vi "环境动力接口交互.vi"   [LabVIEW 2016]
uses:
  PLC/PLC.lvlib
types:
  T1 = cluster{"R0":i16, "R1":i16, "R2":i16, "R3":i16, "R4":i16, "R5":i16, "R6":i16, "R7":i16, "R8":i16, "R9":i16, "R10":i16, "R11":i16, "R12":i16, "R13":i16, "R14":i16, "R15":i16, "R16":i16, "R17":i16, "R18":i16, "R19":i16, "R20":i16, "R21":i16, "R22":i16, "R23":i16, "R24":i16, "R25":i16, "R26":i16, "R27":i16, "R28":i16, "R29":i16, "R30":i16, "R31":i16, "R32":i16, "R33":i16, "R34":i16, "R35":i16, "R36":i16, "R37":i16, "R38":i16, "R39":i16}
  T2 = cluster{"R100":i16, "R101":i16, "R102":i16, "R103":i16, "R104":i16, "R105":i16, "R106":i16, "R107":i16, "R108":i16, "R109":i16, "R110":i16, "R111":i16, "R112":i16, "R113":i16, "R114":i16, "R115":i16, "R116":i16, "R117":i16, "R118":i16, "R119":i16, "R120":i16, "R121":i16, "R122":i16, "R123":i16}
  T3 = cluster{"AD0":sgl, "AD1":sgl, "AD2":sgl, "AD3":sgl, "AD4":sgl, "AD5":sgl}
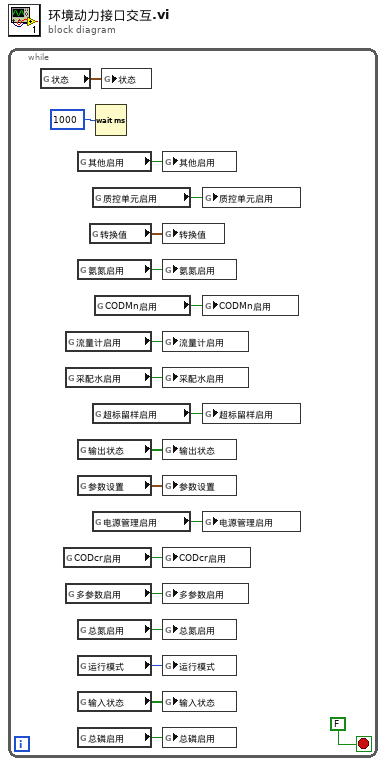
[diagram p0: block diagram]
diagram:
  n1 = while {
    stop <- FALSE stop-if-true
    n2 = global read "采配水全局变量.vi" "状态"() -> (w8:T1)
    n3 = global read "系统设置全局变量.vi" "CODcr启用"() -> (w17:bool)
    n4 = global read "系统设置全局变量.vi" "流量计启用"() -> (w5:bool)
    n5 = global read "系统设置全局变量.vi" "采配水启用"() -> (w15:bool)
    n6 = global read "系统设置全局变量.vi" "多参数启用"() -> (w3:bool)
    n7 = global read "系统设置全局变量.vi" "其他启用"() -> (w4:bool)
    n8 = global read "系统设置全局变量.vi" "氨氮启用"() -> (w16:bool)
    n9 = global read "采配水全局变量.vi" "输出状态"() -> (w20:bool[])
    n10 = global read "采配水全局变量.vi" "参数设置"() -> (w13:T2)
    n11 = global read "系统设置全局变量.vi" "总氮启用"() -> (w11:bool)
    n12 = global read "系统设置全局变量.vi" "运行模式"() -> (w14:enum16{"维护模式", "常规模式", "应急模式", "质控模式"})
    n13 = global read "采配水全局变量.vi" "输入状态"() -> (w19:bool[])
    n14 = global read "系统设置全局变量.vi" "总磷启用"() -> (w10:bool)
    n15 = global read "采配水全局变量.vi" "转换值"() -> (w9:T3)
    n16 = global read "系统设置全局变量.vi" "质控单元启用"() -> (w12:bool)
    n17 = global read "系统设置全局变量.vi" "超标留样启用"() -> (w2:bool)
    n18 = global read "系统设置全局变量.vi" "电源管理启用"() -> (w1:bool)
    n19 = global read "系统设置全局变量.vi" "CODMn启用"() -> (w18:bool)
    n20 = Wait (ms)(milliseconds to wait=u32 1000 ("等待时间（毫秒）")) -> ()  [unwired: 1 out]
    n21 = global write "外部交互全局变量.vi" "状态"(w8) -> ()
    n22 = global write "外部交互全局变量.vi" "其他启用"(w4) -> ()
    n23 = global write "外部交互全局变量.vi" "转换值"(w9) -> ()
    n24 = global write "外部交互全局变量.vi" "氨氮启用"(w16) -> ()
    n25 = global write "外部交互全局变量.vi" "流量计启用"(w5) -> ()
    n26 = global write "外部交互全局变量.vi" "采配水启用"(w15) -> ()
    n27 = global write "外部交互全局变量.vi" "输出状态"(w20) -> ()
    n28 = global write "外部交互全局变量.vi" "参数设置"(w13) -> ()
    n29 = global write "外部交互全局变量.vi" "CODcr启用"(w17) -> ()
    n30 = global write "外部交互全局变量.vi" "多参数启用"(w3) -> ()
    n31 = global write "外部交互全局变量.vi" "总氮启用"(w11) -> ()
    n32 = global write "外部交互全局变量.vi" "运行模式"(w14) -> ()
    n33 = global write "外部交互全局变量.vi" "输入状态"(w19) -> ()
    n34 = global write "外部交互全局变量.vi" "总磷启用"(w10) -> ()
    n35 = global write "外部交互全局变量.vi" "质控单元启用"(w12) -> ()
    n36 = global write "外部交互全局变量.vi" "CODMn启用"(w18) -> ()
    n37 = global write "外部交互全局变量.vi" "超标留样启用"(w2) -> ()
    n38 = global write "外部交互全局变量.vi" "电源管理启用"(w1) -> ()
  }
